vi "Log Event.vi"(0 "TDMS Log In":refnum<class "TDMS Logger.lvclass">, 5 "Group Name (Events)":string="Events", 7 "Channels Names":string[](array[string]), 9 "String Data":string[](array[string]), 11 "Error In":errorcluster) -> (4 "TDMS Log Out":refnum<class "TDMS Logger.lvclass">, 15 "Error Out":errorcluster)   [LabVIEW 2015, in "TDMS Logger.lvlib" / "TDMS Logger.lvclass"]
doc: "Log a 1D array of strings to the TDMS file. Each element corresponds to one event that you want to log to the file. Along with the events that you wire there will be added one Time column, informing about the time of the call of this function.\n\nProviding meaningful names as the channel names is required because they will describe the nature of the logged events."
uses:
  TDMS Logger.lvclass
  TDMS Logger.lvclass/TDMS Logger.ctl
  _Typedefs/Log Action.ctl
  _Typedefs/Log Message.ctl
  _Typedefs/Data Type.ctl
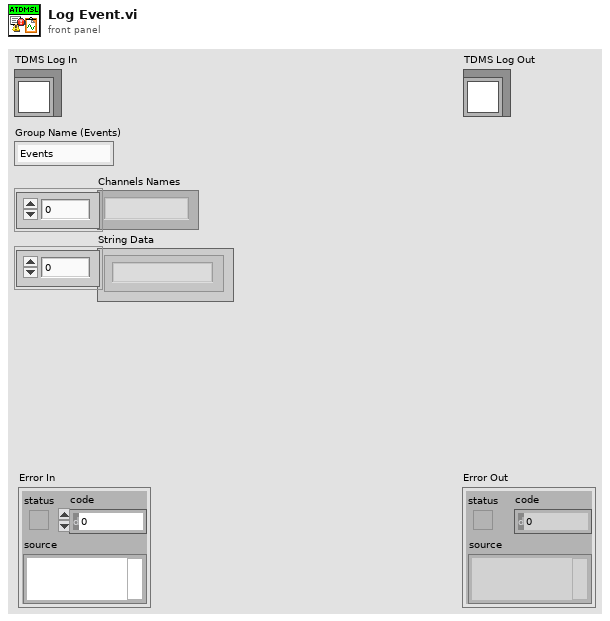
[diagram p1: front panel]
types:
  T1 = typedef "TDMS Logger.lvlib/TDMS Logger.lvclass/Data Type.ctl" = enum16{"I16", "I8", "String", "U16", "U8", "Waveform", "Double", "Single"}
  T2 = typedef "TDMS Logger.lvlib/TDMS Logger.lvclass/Log Message.ctl" = cluster{"Log Action":T3, "Variant":variant, "Data Type":T1, "Group Name":string, "Channels Names":string[]}
  T3 = typedef "TDMS Logger.lvlib/TDMS Logger.lvclass/Log Action.ctl" = enum16{"Handle Old Files", "Status Update", "Stop", "Log Data", "Initialize"}
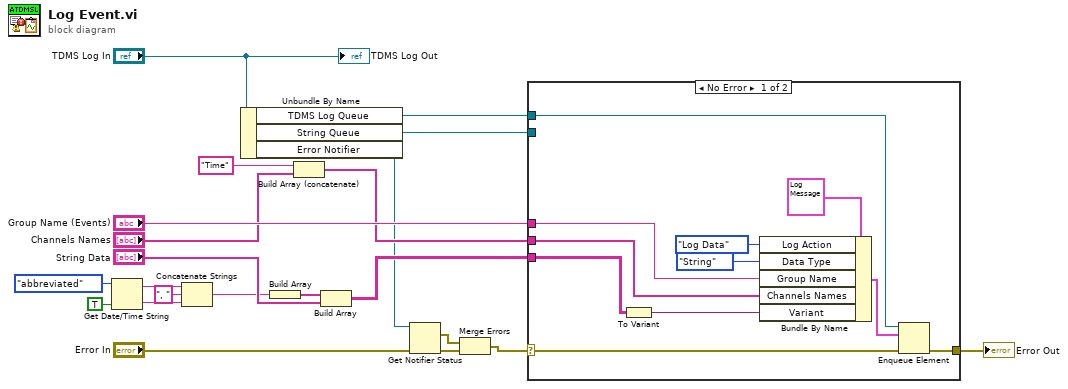
[diagram p0: block diagram]
diagram:
  n1 = Get Date/Time String(date format (0)=enum16{"short", "long", "abbreviated"}."abbreviated", want seconds? (F)=TRUE) -> (date string=w16:string, time string=w15:string)  [unwired: 1 in]
  n2 = Concatenate Strings(w16, ", " ("string"), w15) -> (w13:string)
  n3 = Unbundle By Name("TDMS Log In") -> ("TDMS Log Queue"=w3:refnum<queue>, "String Queue"=w1:refnum<queue>, "Error Notifier"=w9:refnum<notifier>)
  n4 = Build Array(w13) -> (w12:string[])
  n5 = Build Array (concatenate)("Time", "Channels Names") -> (w18:string[])
  n6 = Build Array(w12, "String Data") -> (w11:string[][])
  n7 = Get Notifier Status(notifier=w9, error in (no error)="Error In") -> (current notification=w6:errorcluster, error out=w7:errorcluster)  [unwired: 3 out]
  n8 = Merge Errors(w6, w7) -> (w5:errorcluster)
  n9 = case shown="No Error" w5 {
    selector: w5 -> [w26 w34]
    tunnel: [w25 w34] -> w22
    tunnel: "Group Name (Events)" -> [w28 _]
    tunnel: w18 -> [w27 _]
    tunnel: w11 -> [w24 _]
    tunnel: w3 -> [w29 _]
    tunnel: w1 -> [_ _]
    frame No Error {
      n10 = To Variant(anything=w24) -> (Variant=w23:variant)
      n11 = Bundle By Name(cluster=T2 {"Log Action"=enum."Stop", "Variant"=variant, "Data Type"=enum."String", "Group Name"="", "Channels Names"=[]} ("element"), "Log Action"=Log_Action."Log Data", "Data Type"=Data_Type."String", "Group Name"=w28, "Channels Names"=w27, "Variant"=w23) -> (w32:T2)
      n12 = Enqueue Element(queue=w29, element=w32, error in (no error)=w26) -> (error out=w25:errorcluster)  [unwired: 1 in, 2 out]
    }
    frame Error {
    }
  }
  "Error Out" <- w22
  "TDMS Log Out" <- "TDMS Log In"
